vi "Get App Version.vi"(8 "error in (no error)":errorcluster) -> (0 "error out":errorcluster, 3 "Version":string)   [LabVIEW 2017, in "Application.lvlib" / "Application.lvclass"]
doc: "Retrieves an applications version from the system. If running in LabVIEW, returns \"0.0.0.0\""
uses:
  Application.lvclass
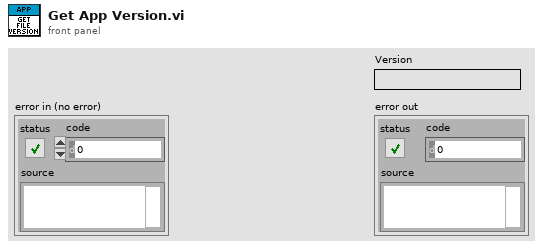
[diagram p1: front panel]
types:
  T1 = enum32{"invalid app kind", "Development System", "Run Time System", "Student Edition", "Embedded LabVIEW", "Evaluation", "Custom"}
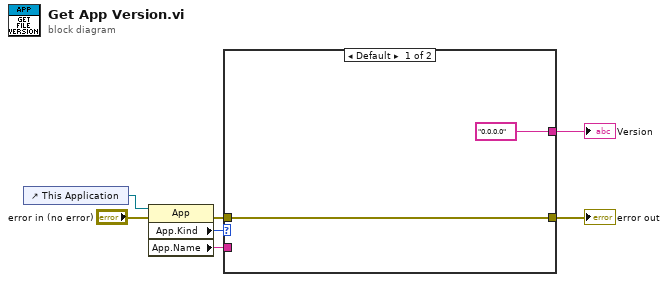
[diagram p0: block diagram]
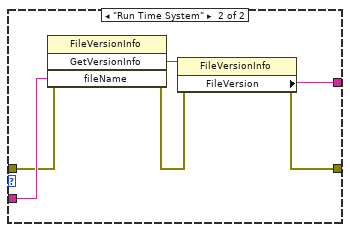
[diagram p2: hidden frame]
diagram:
  n1 = control-ref of="This Application"() -> (w2:refnum<vi>)
  n2 = property class="App"(reference=w2, error in="error in (no error)") -> (error out=w4:errorcluster, "App.Kind"=w5:T1, "App.Name"=w1:string)  [unwired: 1 out]
  n3 = case shown="Default" w5 {
    tunnel: [w9 w13] -> w7
    tunnel: ["0.0.0.0" ("FileVersion") w12] -> w6
    tunnel: w4 -> [w9 w10]
    tunnel: w1 -> [_ w11]
    frame Default {
    }
    frame "Run Time System" {
      n4 = invoke class="FileVersionInfo" method="GetVersionInfo"(error in=w10, "fileName"=w11) -> (error out=w15:errorcluster, "GetVersionInfo"=w14:refnum<k24>)  [unwired: 2 in, 2 out]
      n5 = property class="FileVersionInfo"(reference=w14, error in=w15) -> (error out=w13:errorcluster, "FileVersion"=w12:string)  [unwired: 1 out]
    }
  }
  "Version" <- w6
  "error out" <- w7
